vi "newLVstep.vi"(0 "Engine Reference":refnum<k7>, 5 "Step Name":string, 11 "error in":errorcluster) -> (4 "Engine reference(out)":refnum<k7>, 6 "NewStep (out)":refnum<k7>, 8 "LV Module (out)":refnum<k7>, 15 "error out":errorcluster)   [LabVIEW 2010]
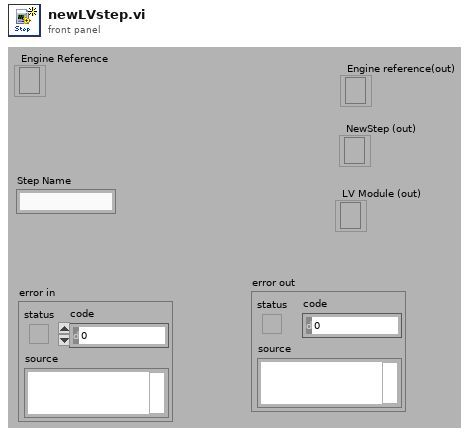
[diagram p1: front panel]
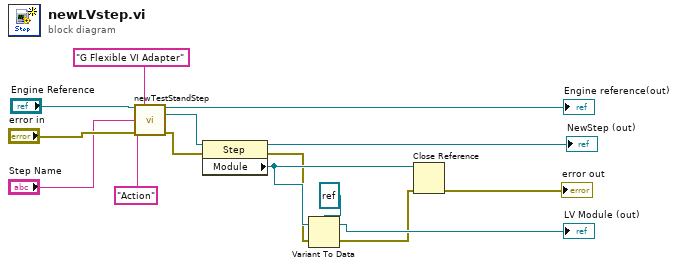
[diagram p0: block diagram]
diagram:
  n1 = call "newTestStandStep.vi"("Engine reference"="Engine Reference", "adapterKeyNameVal"="G Flexible VI Adapter", "stepType"="Action", "Step Name"="Step Name", "error in"="error in") -> ("Engine reference(out)"=→"Engine reference(out)":refnum<k7>, "NewStep (out)"=w9:refnum<k7>, "error out"=w11:errorcluster)  [unwired: 8 in]
  n2 = property class="Step"(reference=w9, error in=w11) -> (reference out=→"NewStep (out)":refnum<k7>, error out=w13:errorcluster, "Module"=w14:refnum<k7>)
  n3 = Variant To Data(error in=w13, Variant=w14, type=refnum<k7> refnum ("Module")) -> (error out=w1:errorcluster, data=→"LV Module (out)":refnum<k7>)
  n4 = Close Reference(reference=w14, error in (no error)=w1) -> (error out=→"error out":errorcluster)
